vi "Init Hardware.vi"(8 "error in (no error)":errorcluster, 11 "ZI Lockin in":refnum<class "ZI Lockin.lvclass">) -> (0 "error out":errorcluster, 3 "ZI Lockin out":refnum<class "ZI Lockin.lvclass">)   [LabVIEW 2016, in "ZI Lockin.lvclass"]
uses:
  ZI Lockin.lvclass
  ZI Lockin.lvclass/ZI Lockin.ctl
  Read Address.vi
  Write ZI Handle.vi
  <instrlib>/Zurich Instruments LabOne/Zurich Instruments LabOne.lvlib
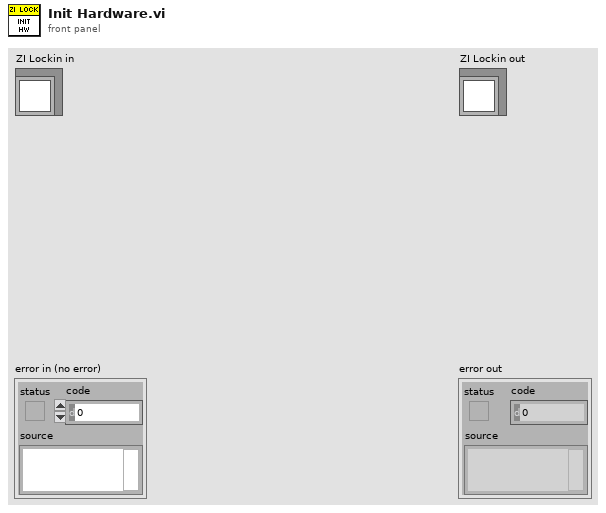
[diagram p1: front panel]
types:
  T1 = typedef "Zurich Instruments LabOne.lvlib/ziTypeHandle.ctl" = cluster{"handleValid":bool, "Conn":u64, "Path Prefix":string, "Handle":u64, "Connected":bool, "Clockbase(s)":dbl}
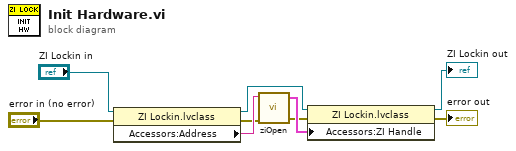
[diagram p0: block diagram]
diagram:
  n1 = property class="ZI Lockin.lvclass"(reference="ZI Lockin in", error in="error in (no error)") -> (reference out=w6:refnum<class "ZI Lockin.lvclass">, error out=w2:errorcluster, "Accessors:Address"=w7:string)
  n2 = call <instrlib>:"ziOpen.vi"("Error In"=w2, "Address"=w7) -> ("Error Out"=w1:errorcluster, "HandleOut"=w3:T1)  [unwired: 2 in, 1 out]
  n3 = property class="ZI Lockin.lvclass"(reference=w6, error in=w1, "Accessors:ZI Handle"=w3) -> (reference out=→"ZI Lockin out":refnum<class "ZI Lockin.lvclass">, error out=→"error out":errorcluster)
